vi "SetMarkerMode.vi"(2 "error in (no error)":errorcluster, 3 "Marker Mode":u8(ring) items=["Fixed Low", "Fixed High", "Automatic", "Replicate Digital 0"], 4 "Marker (0: Marker 1)":u16(ring) items=["Marker 1", "Marker 2", "Marker 3", "Marker 4"], 5 "VISA resource name":refnum<visa-resource-name>) -> (0 "error out":errorcluster, 1 "VISA resource name out":refnum<visa-resource-name>)   [LabVIEW 2020, in "Active Technologies AWG3000.lvlib"]
uses:
  Active Technologies AWG3000.lvlib
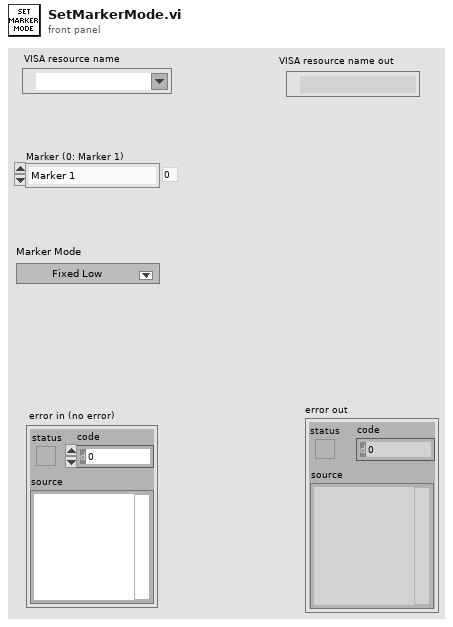
[diagram p1: front panel]
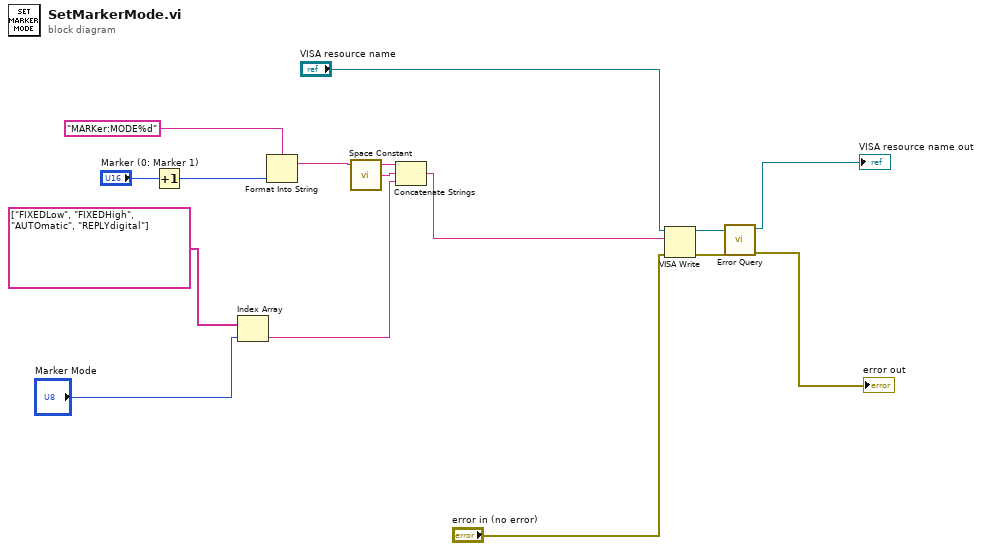
[diagram p0: block diagram]
diagram:
  n1 = Increment(x="Marker (0: Marker 1)") -> (x+1=w7:u16)
  n2 = Index Array(array=string[] ["FIXEDLow", "FIXEDHigh", "AUTOmatic", "REPLYdigital"], index="Marker Mode") -> (element=w1:string)
  n3 = Format Into String(format string="MARKer:MODE%d" ("write buffer"), w7) -> (resulting string=w6:string)  [unwired: 2 in, 1 out]
  n4 = call <vilib>:"Space Constant.vi"() -> ("String"=w5:string)
  n5 = Concatenate Strings(w6, w5, w1) -> (w4:string)
  n6 = VISA Write(VISA resource name="VISA resource name", write buffer=w4, error in (no error)="error in (no error)") -> (VISA resource name out=w13:refnum<visa-resource-name>, error out=w12:errorcluster)  [unwired: 1 out]
  n7 = call "Error Query.vi"("error in (no error)"=w12, "VISA resource name"=w13) -> ("error out"=→"error out":errorcluster, "VISA resource name out"=→"VISA resource name out":refnum<visa-resource-name>)  [unwired: 6 in, 2 out]
